vi "Send Command.vi"(8 "error in (no error)":errorcluster, 11 "Main in":refnum<class "Main.lvclass">) -> (0 "error out":errorcluster, 3 "Main out":refnum<class "Main.lvclass">)   [LabVIEW 2019, in "Main.lvclass"]
doc: "Developed by Kevin Thompson\nkevin@thompsonengineering.net\n\nCopyright 2018\nThompson Engineering, LLC"
uses:
  Main.lvclass
panel:
  in  "CmdData":cluster{"Numeric placeholder":dbl}
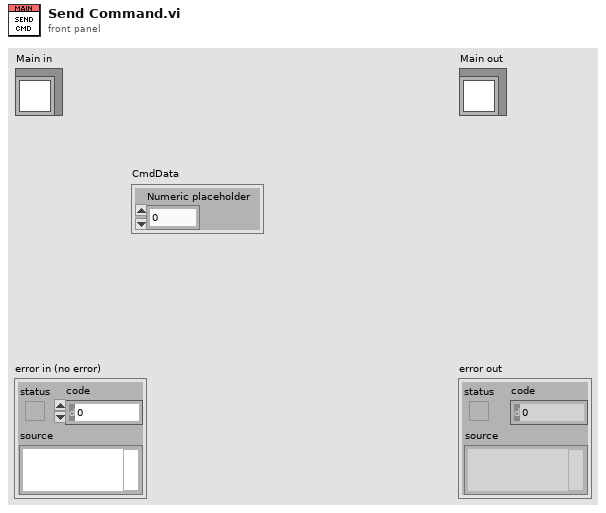
[diagram p1: front panel]
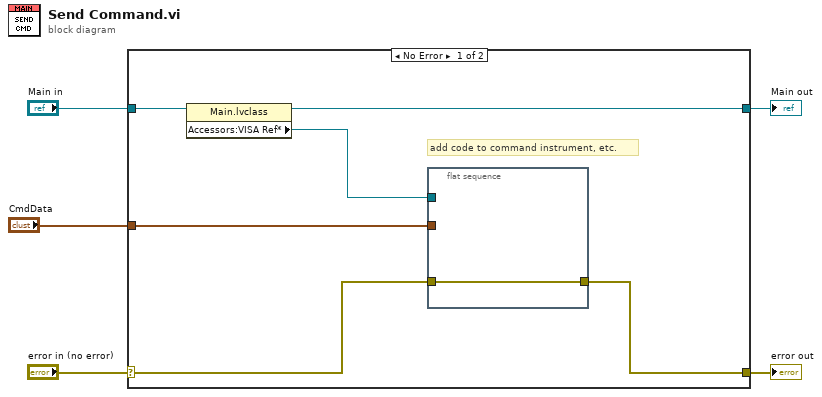
[diagram p0: block diagram]
diagram:
  n1 = case shown="No Error" "error in (no error)" {
    selector: "error in (no error)" -> [w9 w14]
    tunnel: [w8 w14] -> w4
    tunnel: [w10 w13] -> w2
    tunnel: "Main in" -> [w11 w13]
    tunnel: "CmdData" -> [w7 _]
    frame No Error {
      # "add code to command instrument, etc."
      n2 = property class="Main.lvclass"(reference=w11) -> (reference out=w10:refnum<class "Main.lvclass">, "Accessors:VISA Ref*"=w6:refnum<visa-resource-name>)  [unwired: 1 in, 1 out]
      n3 = flat-sequence {
        tunnel: w9 -> [w12]
        tunnel: [w12] -> w8
        tunnel: w7 -> [_]
        tunnel: w6 -> [_]
        frame #0 {
        }
      }
    }
    frame Error {
    }
  }
  "error out" <- w4
  "Main out" <- w2
